vi "EnumToJson.vi"(8 "error in":errorcluster, 10 "Relative Bounds":cluster{"x":i32, "y":i32, "w":i32, "h":i32}, 11 "GObj in":refnum<vi>) -> (0 "error out":errorcluster, 3 "JSON":string)   [LabVIEW 2017]
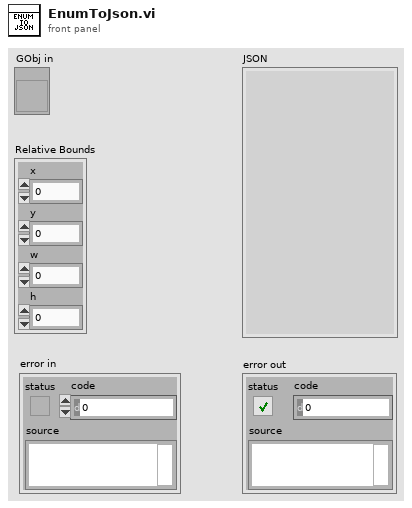
[diagram p1: front panel]
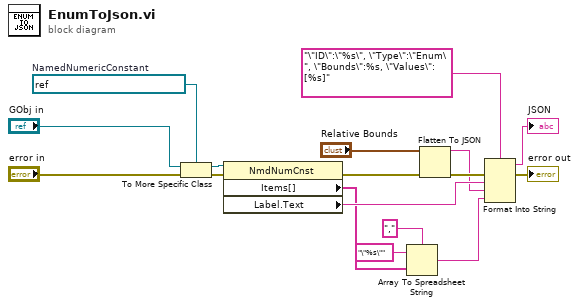
[diagram p0: block diagram]
diagram:
  w17 = refnum<vi> refnum  # NamedNumericConstant
  n1 = To More Specific Class(target class=w17, reference="GObj in", error in="error in") -> (specific class reference=w15:refnum<vi>, error out=w16:errorcluster)
  n2 = property class="NmdNumCnst"(reference=w15, error in=w16) -> (error out=w6:errorcluster, "Items[]"=w10:string[], "Label.Text"=w12:string)  [unwired: 1 out]
  n3 = Array To Spreadsheet String(delimiter (Tab)=",", array=w10, 3:"\"%s\"" ("format string")) -> (spreadsheet string=w11:string)
  n4 = Flatten To JSON(anything="Relative Bounds", error in (no error)=w6) -> (JSON string=w4:string, 11:w5:errorcluster)  [unwired: 1 in]
  n5 = Format Into String(format string="\"ID\":\"%s\", \"Type\":\"Enum\", \"Bounds\":%s, \"Values\": [%s]", error in=w5, w12, w4, w11) -> (resulting string=→"JSON":string, error out=→"error out":errorcluster)  [unwired: 1 in]
